vi "checkBeginNormalGamePlay.vi"(6 "AnyPlayChosen?":bool, 8 "error in (no error)":errorcluster, 11 "NormalGamePlay in":refnum<class "NormalGamePlay.lvclass">) -> (0 "error out":errorcluster, 2 "begin?":bool, 3 "NormalGamePlay out":refnum<class "NormalGamePlay.lvclass">)   [LabVIEW 2021, in "NormalGamePlay.lvclass"]
uses:
  NormalGamePlay.lvclass
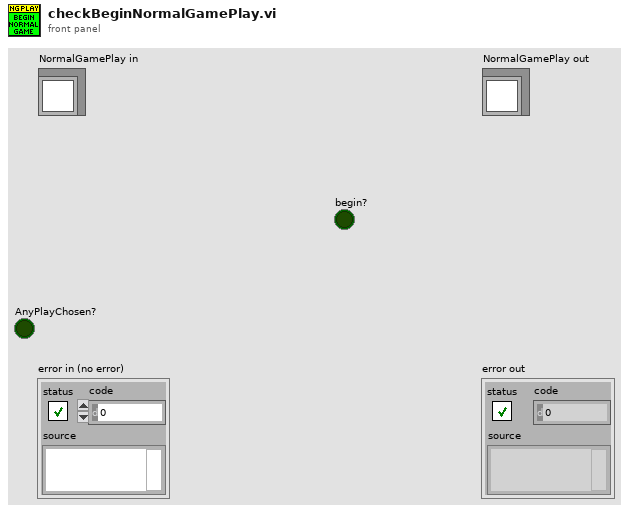
[diagram p1: front panel]
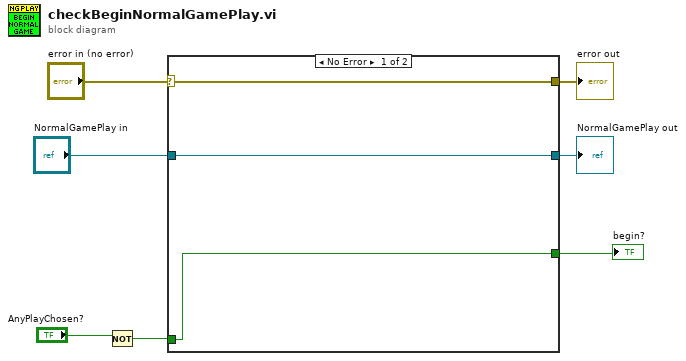
[diagram p0: block diagram]
diagram:
  n1 = Not(x="AnyPlayChosen?") -> (.not. x?=w2:bool)
  n2 = case shown="No Error" "error in (no error)" {
    selector: "error in (no error)" -> [w10 w12]
    tunnel: [w10 w12] -> w6
    tunnel: [w9 w11] -> w4
    tunnel: "NormalGamePlay in" -> [w9 w11]
    tunnel: w2 -> [w8 _]
    tunnel: [w8 _] -> w3
    frame No Error {
    }
    frame Error {
    }
  }
  "error out" <- w6
  "NormalGamePlay out" <- w4
  "begin?" <- w3
